vi "Digital Input DAQ Assistant.vi"() -> ()   [LabVIEW 2020]
panel:
  out "Boolean array":bool[](array[boolean])
  out "data":u32[](array[numeric])
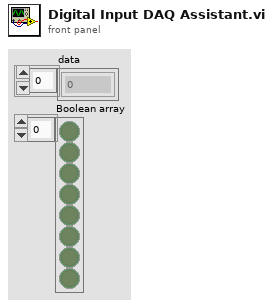
[diagram p1: front panel]
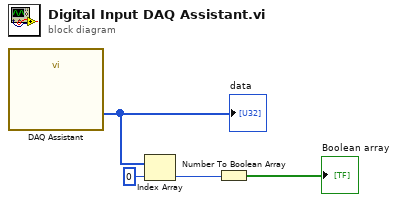
[diagram p0: block diagram]
diagram:
  n1 = call "DAQ Assistant"() -> ("data"=w4:u32[])  [unwired: 17 in, 2 out]
  "data" <- w4
  n2 = Index Array(array=w4, index=0) -> (element=w2:u32)
  n3 = Number To Boolean Array(number=w2) -> (Boolean array=→"Boolean array":bool[])
